vi "set DC test parameters.vi"(7 "DC Parameters":T1={"Voltage Level [V]"=1000, "Hi Limit [A]"=0.005, "Test Time [s] "=3.3, "Dwell Time [s]"=4.4, "Lo Limit [A]"=0.001, "ARC Limit [A]"=0.005, "Ramp Time [s] "=1.1, "Fall Time [s]"=2.2} {"Voltage Level [V]" format="%.3p"; "Hi Limit [A]" format="%#_6p"; "Lo Limit [A]" format="%#_6p"; "ARC Limit [A]" format="%#_6p"}, 8 "error in (no error)":errorcluster, 10 "Step":T2 min=1 max=99 step=1, 11 "VISA Refnum in":refnum<visa-resource-name>) -> (0 "error out":errorcluster, 3 "VISA Refnum out":refnum<visa-resource-name>)   [LabVIEW 2025]
uses:
  Type Def/steps--ring.ctl
  Type Def/AC-DC-IR modes--ring.ctl
  Type Def/AC-DC modes--ring.ctl
  Type Def/DC-IR modes--ring.ctl
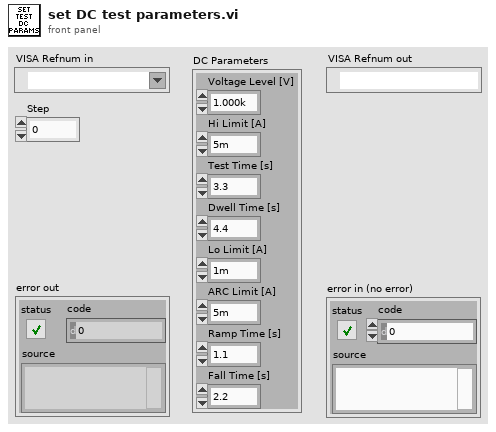
[diagram p1: front panel]
types:
  T1 = cluster{"Voltage Level [V]":u16, "Hi Limit [A]":dbl, "Test Time [s] ":dbl, "Dwell Time [s]":dbl, "Lo Limit [A]":dbl, "ARC Limit [A]":dbl, "Ramp Time [s] ":dbl, "Fall Time [s]":dbl}
  T2 = typedef "steps--ring.ctl" = u8
  T3 = typedef "DC-IR modes--ring.ctl" = u16
  T4 = typedef "AC-DC modes--ring.ctl" = i32
  T5 = typedef "AC-DC-IR modes--ring.ctl" = u16
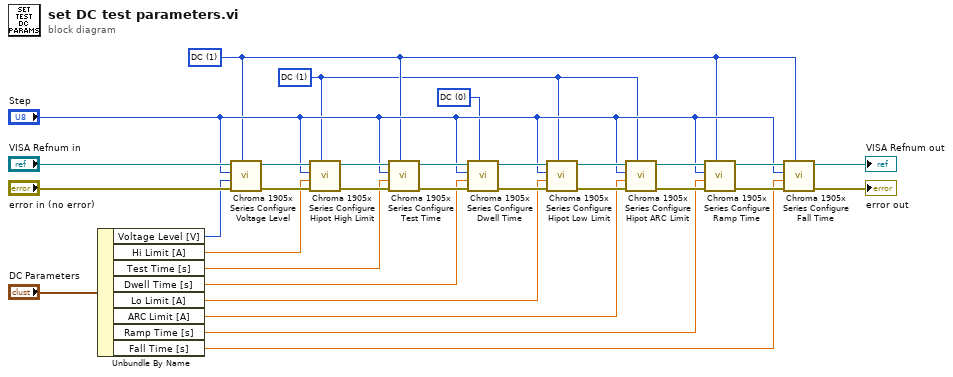
[diagram p0: block diagram]
diagram:
  w12 = T3 0 items=["DC", "IR"] ("Mode")
  w10 = T4 1 items=["AC", "DC"] ("Mode")
  w11 = T5 1 items=["AC", "DC", "IR"] ("Mode")
  n1 = Unbundle By Name("DC Parameters") -> ("Voltage Level [V]"=w8:u16, "Hi Limit [A]"=w7:dbl, "Test Time [s]"=w6:dbl, "Dwell Time [s]"=w5:dbl, "Lo Limit [A]"=w4:dbl, "ARC Limit [A]"=w3:dbl, "Ramp Time [s]"=w2:dbl, "Fall Time [s]"=w1:dbl)
  n2 = call "Chroma 1905x Series Configure Voltage Level.vi"("Mode"=w11, "error in (no error)"="error in (no error)", "Voltage Level [V]"=w8, "Step"="Step", "VISA resource name"="VISA Refnum in") -> ("error out"=w20:errorcluster, "VISA resource name out"=w17:refnum<visa-resource-name>)  [unwired: 5 in]
  n3 = call "Chroma 1905x Series Configure Hipot High Limit.vi"("Mode"=w10, "error in (no error)"=w20, "Hi Limit [A]"=w7, "Step"="Step", "VISA resource name"=w17) -> ("error out"=w27:errorcluster, "VISA resource name out"=w28:refnum<visa-resource-name>)  [unwired: 5 in]
  n4 = call "Chroma 1905x Series Configure Test Time.vi"("Mode"=w11, "error in (no error)"=w27, "Test Time [s]"=w6, "Step"="Step", "VISA resource name"=w28) -> ("error out"=w30:errorcluster, "VISA resource name out"=w14:refnum<visa-resource-name>)  [unwired: 5 in]
  n5 = call "Chroma 1905x Series Configure Dwell Time.vi"("Mode"=w12, "error in (no error)"=w30, "Dwell Time [s]"=w5, "Step"="Step", "VISA resource name"=w14) -> ("error out"=w29:errorcluster, "VISA resource name out"=w31:refnum<visa-resource-name>)  [unwired: 5 in]
  n6 = call "Chroma 1905x Series Configure Hipot Low Limit.vi"("Mode"=w10, "error in (no error)"=w29, "Lo Limit [A]"=w4, "Step"="Step", "VISA resource name"=w31) -> ("error out"=w21:errorcluster, "VISA resource name out"=w22:refnum<visa-resource-name>)  [unwired: 5 in]
  n7 = call "Chroma 1905x Series Configure Hipot ARC Limit.vi"("Mode"=w10, "error in (no error)"=w21, "ARC Limit [A]"=w3, "Step"="Step", "VISA resource name"=w22) -> ("error out"=w23:errorcluster, "VISA resource name out"=w25:refnum<visa-resource-name>)  [unwired: 5 in]
  n8 = call "Chroma 1905x Series Configure Ramp Time.vi"("Mode"=w11, "error in (no error)"=w23, "Ramp Time [s]"=w2, "Step"="Step", "VISA resource name"=w25) -> ("error out"=w24:errorcluster, "VISA resource name out"=w26:refnum<visa-resource-name>)  [unwired: 5 in]
  n9 = call "Chroma 1905x Series Configure Fall Time.vi"("Mode"=w11, "error in (no error)"=w24, "Fall Time [s]"=w1, "Step"="Step", "VISA resource name"=w26) -> ("error out"=→"error out":errorcluster, "VISA resource name out"=→"VISA Refnum out":refnum<visa-resource-name>)  [unwired: 5 in]
